vi "Zadanie 3.vi"() -> ()   [LabVIEW 2020]
panel:
  out "number":u32
  out "Array":bool[](array[boolean])
  in  "CP":bool
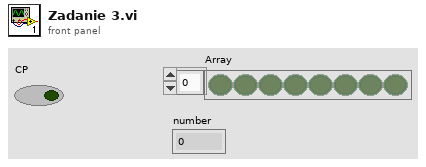
[diagram p1: front panel]
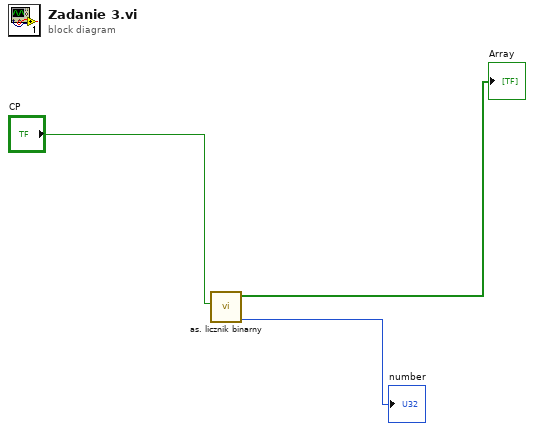
[diagram p0: block diagram]
diagram:
  n1 = call "as. licznik binarny.vi"("CP"="CP") -> ("iloœæ zliczeñ"=→"number":u32, "Tablica zliczeñ"=→"Array":bool[])  [unwired: 9 in]
